vi "RAW TO INTIGER.vi"(11 "data in":string) -> (2 "SGL":sgl, 3 "INITEER":u16[](array[numeric]))   [LabVIEW 2023]
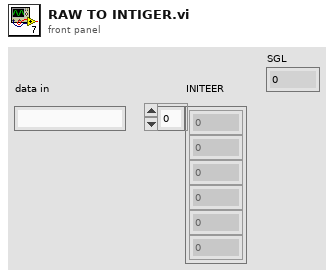
[diagram p1: front panel]
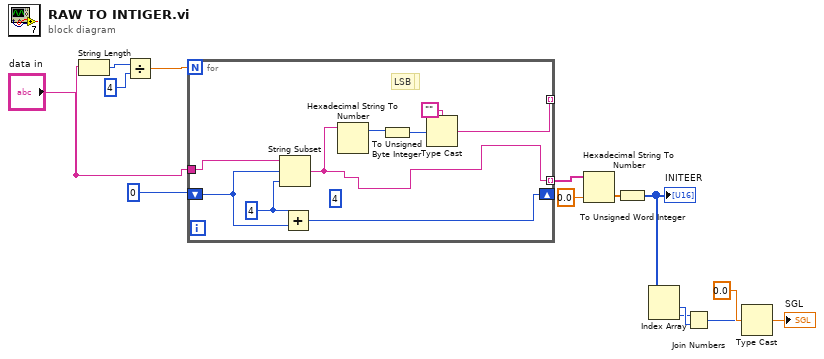
[diagram p0: block diagram]
diagram:
  n1 = String Length(string="data in") -> (length=w12:i32)
  n2 = Divide(x=w12, y=4) -> (x/y=w9:dbl)
  n3 = for {
    N: w9 -> [_]
    tunnel: "data in" -> [w23]
    shift-right: [w22] -> _
    shift-left: 0 ("length (rest)") -> [w21]
    tunnel: [w19] -> w7 mode=indexing
    tunnel: [w16] -> _ mode=indexing
    (unwired) 4 ("length (rest)")
    w20 = 4 ("x")
    # "LSB"
    # "MSB"
    n4 = String Subset(string=w23, offset (0)=w21, length (rest)=w20) -> (substring=w19:string)
    n5 = Add(x=w20, y=w21) -> (x+y=w22:i32)
    n6 = Hexadecimal String To Number(string=w19) -> (offset past number=w18:i32)  [unwired: 2 in, 1 out]
    n7 = To Unsigned Byte Integer(number=w18) -> (unsigned 8bit integer=w17:u8)
    n8 = Type Cast(type="", x=w17) -> (*(type *) &x=w16:string)
  }
  n9 = Hexadecimal String To Number(string=w7, default (0uL)=0.0 ("default (0 U32)")) -> (number=w13:dbl[])  [unwired: 1 in, 1 out]
  n10 = To Unsigned Word Integer(number=w13) -> (unsigned 16bit integer=w2:u16[])
  "INITEER" <- w2
  n11 = Index Array(array=w2) -> (element #1=w5:u16, element #2=w4:u16)  [unwired: 2 in]
  n12 = Join Numbers(hi=w4, lo=w5) -> ((hi.lo)=w3:u32)
  n13 = Type Cast(type=sgl 0.0 ("default (0 U32)"), x=w3) -> (*(type *) &x=→"SGL":sgl)
